vi "HAL_Configure Channel.vi"(8 "error in":errorcluster, 10 "Channel ID":string, 11 "Handle In":T1) -> (0 "error out":errorcluster, 3 "Handle Out":T1)   [LabVIEW 2015]
uses:
  Handle.ctl
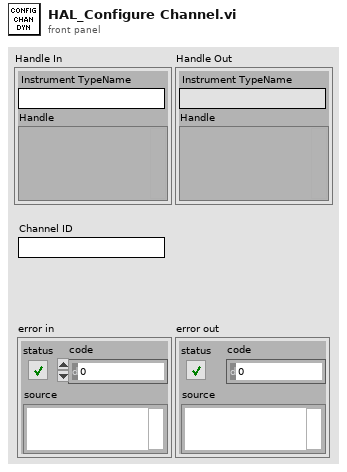
[diagram p1: front panel]
types:
  T1 = typedef "Handle.ctl" = cluster{"Instrument TypeName":string, "Handle":variant}
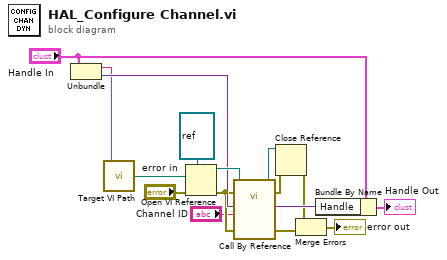
[diagram p0: block diagram]
diagram:
  n1 = Unbundle("Handle In") -> ("Instrument TypeName"=w7:string, "Handle"=w14:variant)
  n2 = call "Target VI Path.vi"("Instrument Name"=w7) -> ("Path to VI"=w8:path)
  n3 = Open VI Reference(type specifier VI Refnum (for type only)=refnum<vi> refnum, vi path=w8, error in (no error)="error in") -> (vi reference=w15:refnum<vi>, error out=w5:errorcluster)  [unwired: 3 in]
  n4 = call-by-ref "?"(reference=w15, error in=w5, "error in"=w5, "Channel ID"="Channel ID", "Handle In"=w14) -> (reference out=w4:refnum<vi>, error out=w2:errorcluster, 0:"error out"=w10:errorcluster, "Handle Out"=w12:variant)  [unwired: 7 in]
  n5 = Close Reference(reference=w4, error in (no error)=w2) -> (error out=w1:errorcluster)
  n6 = Merge Errors(w1, w10) -> (→"error out":errorcluster)
  n7 = Bundle By Name(cluster="Handle In", "Handle"=w12) -> (→"Handle Out":T1)
